vi "State Machine(8.1).vi"() -> ()   [LabVIEW 2014]
uses:
  State Enum.ctl
panel:
  in  "Menu":T1
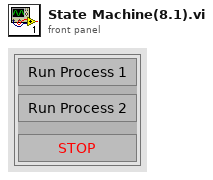
[diagram p1: front panel]
types:
  T1 = cluster{"Process 1":bool, "Process 2":bool, "stop":bool}
  T2 = typedef "State Enum.ctl" = enum32{"Idle", "Process 1", "Process 2", "Stop"}
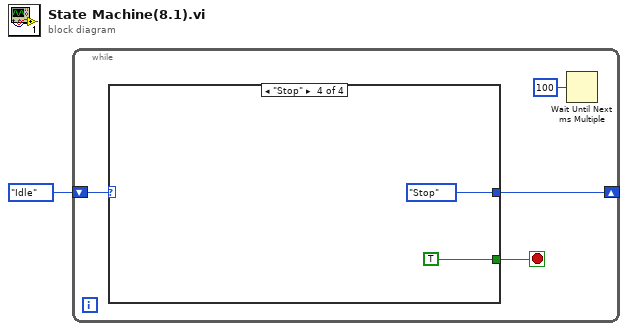
[diagram p0: block diagram]
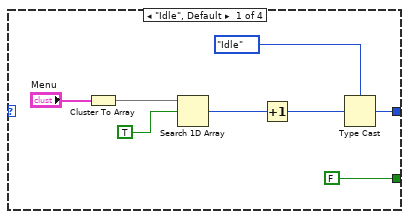
[diagram p2: hidden frame]
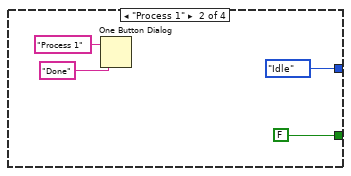
[diagram p3: hidden frame]
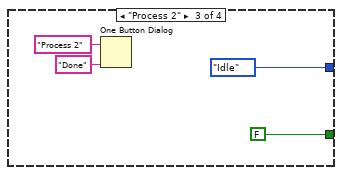
[diagram p4: hidden frame]
diagram:
  n1 = while {
    shift-right: [w3] -> _
    shift-left: State_Enum."Idle" -> [w5]
    stop <- w2 stop-if-true
    n2 = case shown="\"Stop\"" w5 {
      tunnel: [w7 State_Enum."Idle" State_Enum."Idle" State_Enum."Stop"] -> w3
      tunnel: [FALSE ("element") FALSE ("element") FALSE ("element") TRUE ("element")] -> w2
      frame "Idle", Default {
        n3 = Cluster To Array(cluster="Menu") -> (array=w12:bool[])
        n4 = Search 1D Array(1D array=w12, element=TRUE) -> (index of element=w10:i32)  [unwired: 1 in]
        n5 = Increment(x=w10) -> (x+1=w9:i32)
        n6 = Type Cast(type=State_Enum."Idle", x=w9) -> (*(type *) &x=w7:T2)
      }
      frame "Process 1" {
        n7 = One Button Dialog(message="Process 1", button name ("OK")="Done") -> ()  [unwired: 1 out]
      }
      frame "Process 2" {
        n8 = One Button Dialog(message="Process 2", button name ("OK")="Done") -> ()  [unwired: 1 out]
      }
      frame "Stop" {
      }
    }
    n9 = Wait Until Next ms Multiple(millisecond multiple=u32 100) -> ()  [unwired: 1 out]
  }
